vi "Configure Data Length.vi"(8 "error in (no error)":errorcluster, 10 "Data Length":i32=10000, 11 "Debug Log In":refnum<class "Debug Log.lvclass">) -> (0 "error out":errorcluster, 3 "Debug Log Out":refnum<class "Debug Log.lvclass">)   [LabVIEW 2020, in "Debug Log.lvclass"]
uses:
  Debug Log.lvclass
  Debug Log.lvclass/Debug Log.ctl
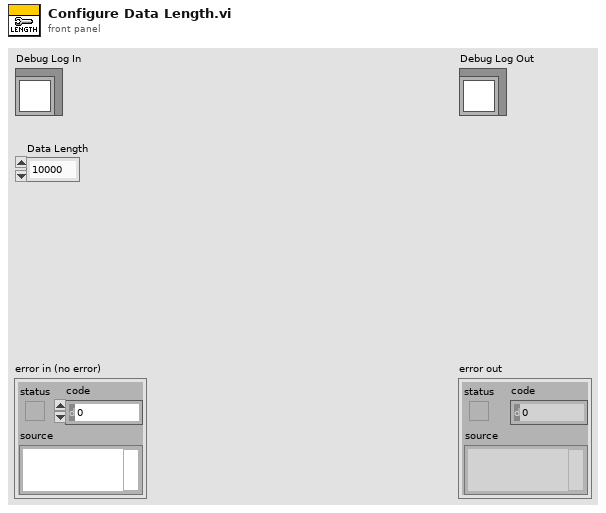
[diagram p1: front panel]
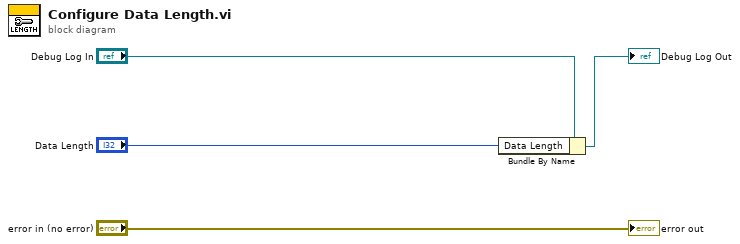
[diagram p0: block diagram]
diagram:
  n1 = Bundle By Name(cluster="Debug Log In", "Data Length"="Data Length") -> (→"Debug Log Out":refnum<class "Debug Log.lvclass">)
  "error out" <- "error in (no error)"
